vi "Publish.vi"   [LabVIEW 2014, in "FrontPanelPublisher.lvlib"]
uses:
  FrontPanelPublisher.lvlib
  FrontPanelManager_class/Controls/WebsocketInfo.ctl
  WebFrontPanel_class/WebFrontPanel.lvclass
  FrontPanelManager_class/FrontPanelManager.lvclass
types:
  T1 = typedef "FrontPanelPublisher.lvlib/FrontPanelManager.lvclass/WebsocketInfo.ctl" = cluster{"Hostname":string, "Port":u16}
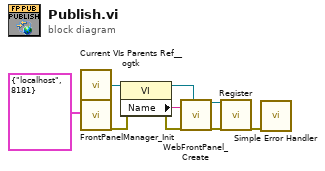
[diagram p0: block diagram]
diagram:
  n1 = call <userlib>:"Current VIs Parents Ref__ogtk.vi"() -> ("Calling VI's Reference"=w6:refnum<vi>)  [unwired: 2 in]
  n2 = call "FrontPanelManager_Init.vi"("Websocket Info"=T1 {"Hostname"="localhost", "Port"=8181}) -> ("error out"=w4:errorcluster)  [unwired: 17 in, 1 out]
  n3 = property class="VI"(reference=w6, error in=w4) -> (reference out=w5:refnum<vi>, error out=w3:errorcluster, "Name"=w9:string)
  n4 = call "WebFrontPanel_Create.vi"("VI Name"=w9, "error in (no error)"=w3, "VI Reference"=w5) -> ("reference out"=w7:refnum<class "WebFrontPanel.lvclass">, "error out"=w8:errorcluster)  [unwired: 15 in]
  n5 = call "Register.vi"("WebFrontPanel"=w7, "error in (no error)"=w8) -> ("error out"=w2:errorcluster)  [unwired: 17 in]
  n6 = call <vilib>:"Simple Error Handler.vi"("error in (no error)"=w2) -> ()  [unwired: 4 in, 5 out]
